vi "DataU16组合.vi"(10 "高字节":u8, 11 "低字节":u8) -> (3 "数值输出":u16)   [LabVIEW 2016]
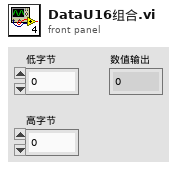
[diagram p1: front panel]
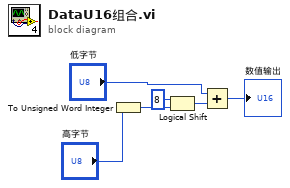
[diagram p0: block diagram]
diagram:
  n1 = To Unsigned Word Integer(number="高字节") -> (unsigned 16bit integer=w3:u16)
  n2 = Logical Shift(y=i16 8, x=w3) -> (x << y=w4:u16)
  n3 = Add(x="低字节", y=w4) -> (x+y=→"数值输出":u16)
